vi "TracePoint.vi"() -> (3 "template trace point":string)   [LabVIEW 2017, in "ModbusMaster.lvlib"]
uses:
  <vilib>/addons/InsightCM/Devices/Shared/Common/ModbusMaster/ModbusMaster.lvlib
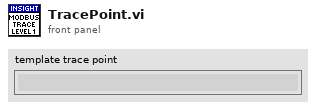
[diagram p1: front panel]
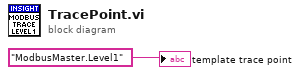
[diagram p0: block diagram]
diagram:
  "template trace point" <- "ModbusMaster.Level1" ("ProcessName")
